vi "FLIN Write Data.vi"(6 "Len":u32, 7 "pData":u8[](array[numeric])=array[4097 elements], 9 "Flags":u8, 10 "LINIndex":u8, 11 "DevHandle":i32) -> (3 "function return":i32, 5 "pData out":u8[](array[numeric]))   [LabVIEW 2010, in "usb2fast_lin.lvlib"]
doc: "int WINAPI FLIN_WriteData(int DevHandle,unsigned char LINIndex,unsigned char Flags,unsigned char *pData,unsigned int Len);"
uses:
  usb2fast_lin.lvlib
  USB2XXX/trunk/USB2XXX/USB2XXX/vs2010/Release/USB2XXX.dll
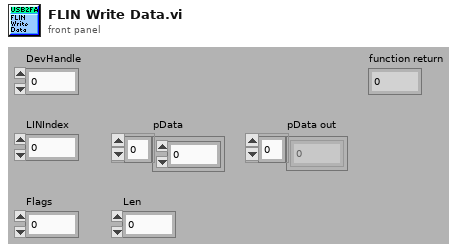
[diagram p1: front panel]
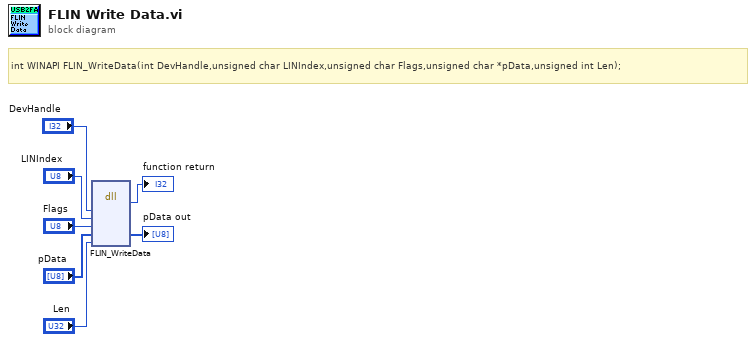
[diagram p0: block diagram]
diagram:
  # "int WINAPI FLIN_WriteData(int DevHandle,unsigned char LINIndex,unsigned char Flags,unsigned char *pData,unsigned int Len);"
  n1 = dll-call lib="E:/Projects/USB2XXX/trunk/USB2XXX/USB2XXX/vs2010/Release/USB2XXX.*" fn="FLIN_WriteData"("DevHandle"="DevHandle", "LINIndex"="LINIndex", "Flags"="Flags", "pData"="pData", "Len"="Len") -> (→"function return":i32, "pData"=→"pData out":u8[])  [unwired: 7 in, 2 out]
